vi "SetConfig.vi"(8 "error in (no error)":errorcluster, 10 "Variant":variant, 11 "StandardFunction in":refnum<class "StandardFunction.lvclass">) -> (0 "error out":errorcluster, 3 "StandardFunction out":refnum<class "StandardFunction.lvclass">)   [LabVIEW 2014, in "Functions.lvlib" / "StandardFunction.lvclass"]
uses:
  StandardFunction.lvclass
  TypeDefs/StdWfrms.ctl
  TypeDefs/StdWfrm.ctl
  StandardFunction.lvclass/StandardFunction.ctl
  Accessors/Write StandardWfrms.vi
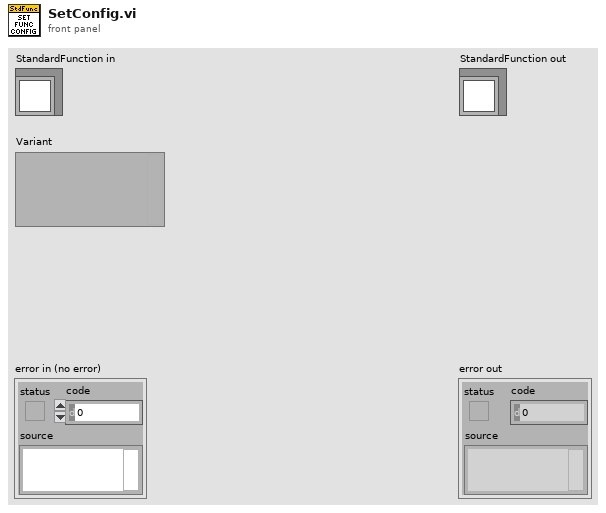
[diagram p1: front panel]
types:
  T1 = typedef "Functions.lvlib/StandardFunction.lvclass/StdWfrms.ctl" = cluster{"Count":u16, "StandardWfrm":T2[]}
  T2 = typedef "Functions.lvlib/StandardFunction.lvclass/StdWfrm.ctl" = cluster{"Amplitude":dbl, "DcOffset":dbl, "DutyCycle":dbl, "Frequency":dbl, "Phase":dbl, "Waveform":enum16{"Sine", "Square", "Triangle", "Ramp Up", "Ramp Down", "DC"}, "Handle":string}
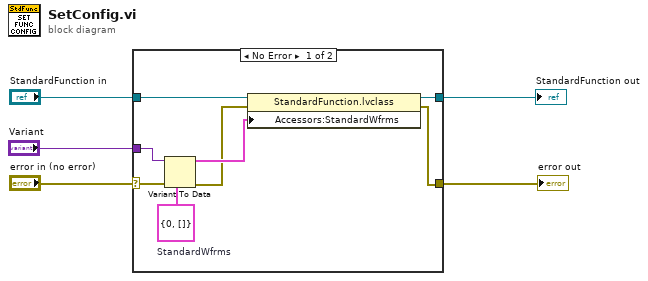
[diagram p0: block diagram]
diagram:
  n1 = case shown="No Error" "error in (no error)" {
    selector: "error in (no error)" -> [w13 w15]
    tunnel: "StandardFunction in" -> [w10 w14]
    tunnel: "Variant" -> [w12 _]
    tunnel: [w6 w15] -> w2
    tunnel: [w7 w14] -> w1
    frame No Error {
      w11 = T1 {"Count"=0, "StandardWfrm"=[]}  # StandardWfrms
      n2 = Variant To Data(error in=w13, type=w11, Variant=w12) -> (data=w9:T1, error out=w8:errorcluster)
      n3 = property class="StandardFunction.lvclass"(reference=w10, error in=w8, "Accessors:StandardWfrms"=w9) -> (reference out=w7:refnum<class "StandardFunction.lvclass">, error out=w6:errorcluster)
    }
    frame Error {
    }
  }
  "error out" <- w2
  "StandardFunction out" <- w1
